vi "SimpleExample Asynchronous Query.vi"() -> ()   [LabVIEW 2011]
uses:
  Interprocess Messenger/QueueMessenger/QueueMessenger.lvclass
  Interprocess Messenger/TextVarientMessage/MSG.lvclass
  Interprocess Messenger/Send/Send.lvclass
  Interprocess Messenger/Send/Send (no data).vi
  Interprocess Messenger/TextVarientMessage/Reply (varient).vi
  Interprocess Messenger/EventMessenger/EventMessenger.lvclass
  Interprocess Messenger/VarMessage/Extract Varient (static).vi
  Interprocess Messenger/TextVarientMessage/Write (no data).vi
  Interprocess Messenger/Send/Send Message.vi
panel:
  out "Time":timestamp
  # "Any Key Down to stop"
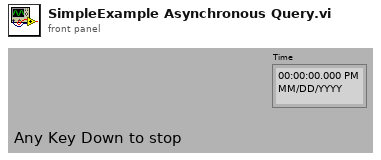
[diagram p1: front panel]
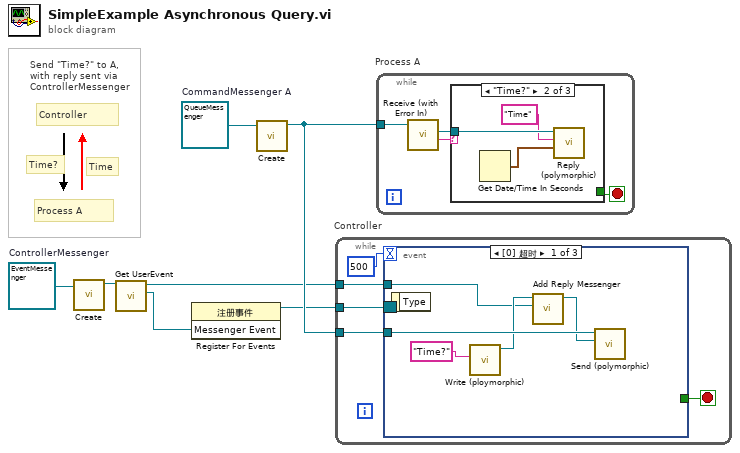
[diagram p0: block diagram]
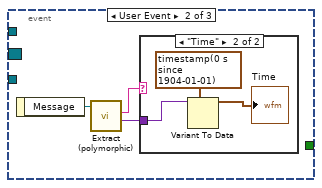
[diagram p2: hidden frame]
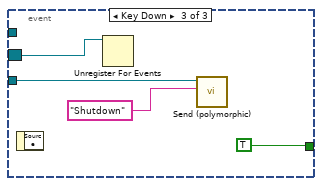
[diagram p4: hidden frame]
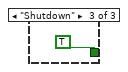
[diagram p6: hidden frame]
diagram:
  w5 = refnum<class "EventMessenger.lvclass"> refnum  # ControllerMessenger
  w7 = refnum<class "QueueMessenger.lvclass"> refnum  # CommandMessenger A
  # "Send \"Time?\" to A, \nwith reply sent via \nControllerMessenger"
  # "Time"
  # "Time?"
  # "Process A"
  # "Controller"
  n1 = call-dynamic "Create.vi"("EventMessenger in"=w5) -> ("EventMessenger out"=w4:refnum<class "EventMessenger.lvclass">)  [unwired: 1 in, 9 out]
  n2 = call-dynamic "Get UserEvent.vi"("EventMessenger"=w4) -> ("Messenger Event"=w3:refnum<user-event>, "EventMessenger out"=w1:refnum<class "EventMessenger.lvclass">)  [unwired: 1 in, 8 out]
  n3 = register-events(w3) -> (reference out=w2:refnum<event-registration>)  [unwired: 2 in, 1 out]
  n4 = call-dynamic "Create.vi"("QueueMessenger in"=w7) -> ("QueueMessenger out"=w6:refnum<class "QueueMessenger.lvclass">)  [unwired: 1 in, 9 out]
  n5 = while "Controller" {
    tunnel: w6 -> [w12]
    tunnel: w2 -> [w9]
    tunnel: w1 -> [w8]
    stop <- w11 stop-if-true
    n6 = event shown="[0] 超时" {
      selector: w9 -> [_ _ w24]
      dyn-events: _ -> [_ _ _]
      timeout: 500 -> [_ _ _]
      tunnel: w12 -> [w17 _ w26]
      tunnel: [_ _ TRUE] -> w11
      tunnel: w8 -> [w14 _ _]
      event Timeout {
        n7 = event-data() -> ()  [unwired: 2 out]
        n8 = call-poly "Write (ploymorphic).vi"("Label"="Time?") -> ("Message"=w15:refnum<class "MSG.lvclass">)  [unwired: 1 in, 9 out]
        n9 = call "Add Reply Messenger.vi"("Reply to..."=w14, "Message"=w15) -> ("Message"=w13:refnum<class "MSG.lvclass">)  [unwired: 1 in, 8 out]
        n10 = call-poly "Send (polymorphic).vi"("Message"=w13, "MSR Parent in"=w17) -> ()  [unwired: 1 in, 9 out]
      }
      event User Event {
        n11 = event-data() -> ("Message"=w20:refnum<class "MSG.lvclass">)  [unwired: 1 out]
        n12 = call-poly "Extract (polymorphic).vi"("Interprocess Message in"=w20) -> ("Varient"=w19:variant, "Label"=w18:string)  [unwired: 1 in, 8 out]
        n13 = case shown="\"Time\"" w18 {
          tunnel: w19 -> [_ w21]
          frame Default {
          }
          frame "Time" {
            n14 = Variant To Data(type=timestamp(0 s since 1904-01-01) ("current time"), Variant=w21) -> (data=→"Time":timestamp)  [unwired: 1 in, 1 out]
          }
        }
      }
      event Key Down {
        n15 = event-data() -> ()  [unwired: 2 out]
        n16 = Unregister For Events(event registration refnum=w24) -> ()  [unwired: 1 in, 1 out]
        n17 = call-poly "Send (polymorphic).vi"("Label"="Shutdown", "MSR Parent in"=w26) -> ()  [unwired: 1 in, 9 out]
      }
    }
  }
  n18 = while "Process A" {
    tunnel: w6 -> [w31]
    stop <- w28 stop-if-true
    n19 = call-dynamic "Receive (with Error In).vi"("MGR in"=w31) -> ("Label"=w30:string, "Message"=w29:refnum<class "MSG.lvclass">)  [unwired: 2 in, 7 out]
    n20 = case shown="\"Time?\"" w30 {
      tunnel: w29 -> [_ w34 _]
      tunnel: [_ _ TRUE] -> w28
      frame "False", Default {
      }
      frame "Time?" {
        n21 = Get Date/Time In Seconds() -> (seconds since 1Jan1904=w33:timestamp)
        n22 = call-poly "Reply (polymorphic).vi"("Varient"=w33, "Reply"="Time", "Message to Reply to"=w34) -> ()  [unwired: 1 in, 8 out]
      }
      frame "Shutdown" {
      }
    }
  }
